vi "BLEGUI.vi"() -> ()   [LabVIEW 2019]
doc: "This example performs writes and reads on a serial port, as directed by the user. You can press the Write and Read buttons, and change the Read Count, while the example is running.\n\nThe parameters set for the serial port must match the parameters of the connected instrument or device. In this example, the Read Count parameter specifies the number of bytes that the serial port reads. If there were more bytes at the port than the specified number, those bytes would not be read. If there were less bytes at the port than the specified number, you would receive a timeout error.\n\nThis example expands upon the flow control options for XON and XOFF, allowing the user to choose those control characters. Also, the user can enable or disable a termination character. Some devices require a termination character in order to identify the end of command strings. Some devices send a termination character to signify the end of data to be read. This example shows how you can end the Read operation once a termination character is detected in the buffer and/or append a termination character at the end of the Write data."
uses:
  Serial - Settings.ctl
  Serial - XON-XOFF Characters.ctl
  Serial - ASCII Characters.ctl
  <vilib>/Instr/_visa.llb/VISA Configure Serial Port (Instr).vi
panel:
  in  "Stop":bool
  in  "Termination Character":u8=10 format="%.0x"
  in  "End Write on Termination Character?":bool=TRUE
  in  "XON/XOFF Characters":T1={"XON"=enum."DC1", "XOFF"=enum."DC3"}
  in  "Serial Settings":T3={"baud rate"=9600, "data bits"=8, "parity"=enum."None", "stop bits"=10, "flow control"=0} {"flow control" items=["None"=0, "XON/XOFF"=1, "RTS/CTS"=2, "DTR/DSR"=4]; "stop bits" items=["1.0"=10, "1.5"=15, "2.0"=20]; "data bits" min=5 max=8 step=1; "baud rate" items=["75"=75, "110"=110, "134"=134, "150"=150, "300"=300, "600"=600, "1200"=1200, "1800"=1800, "2400"=2400, "4800"=4800, "7200"=7200, "9600"=9600, "14400"=14400, "19200"=19200, "28800"=28800, "38400"=38400, "56000"=56000, "57600"=57600, "115200"=115200, "128000"=128000, "230400"=230400]}
  in  "End Read on Termination Character?":bool=TRUE
  in  "VISA resource name":refnum<visa-resource-name>="COM1"
  in  "Read Count":u32=1000
  out "Response":string
  out "Gyro":T4(graph)
  out "Acc":T4(graph)
  out "W4":dbl
  out "W3":dbl
  out "W2":dbl
  out "W1":dbl
  out "GZ":dbl
  out "GY":dbl
  out "GX":dbl
  out "Z":dbl
  out "Y":dbl
  out "X":dbl
  out "Z":dbl(slide) scale=0.0..2.0
  out "Y":dbl(slide) scale=-1.0..1.0
  out "X":dbl(slide) scale=-1.0..1.0
  out "Roll (deg)":dbl(knob) scale=-180.0..180.0
  out "Pitch (deg)":dbl(knob) scale=-90.0..90.0
  in  "Activate Drone Location":bool
  out "Distance 2 (mm)":i32
  out "Ultrasonic 2":dbl(knob) scale=0.0..300.0
  out "Ultrasonic 1":dbl(knob) scale=0.0..300.0
  out "Distance 1 (mm)":i32
  in  "Quick Command":string="*IDN?"
  in  "Command QuadCopter":bool
  in  "Down":bool
  in  "Up":bool
  in  "Left":bool
  in  "Right":bool
  in  "STOP Quadcopter":bool
  # "SERIAL SETTINGS"
  # "0xA is equivalent to a '\\n' character, which is a line feed."
  # "STATUS & CONTINUOUS FEED"
  # "QUADCOPTER & MOTORS"
  # "ON"
  # "OFF"
  # "Speed of Motors (deg s-1)"
  # "Gyro (deg s-1)"
  # "Acc (G)"
  # "MOTION SENSING"
  # "COMMAND QUADCOPTER"
  # "ON"
  # "OFF"
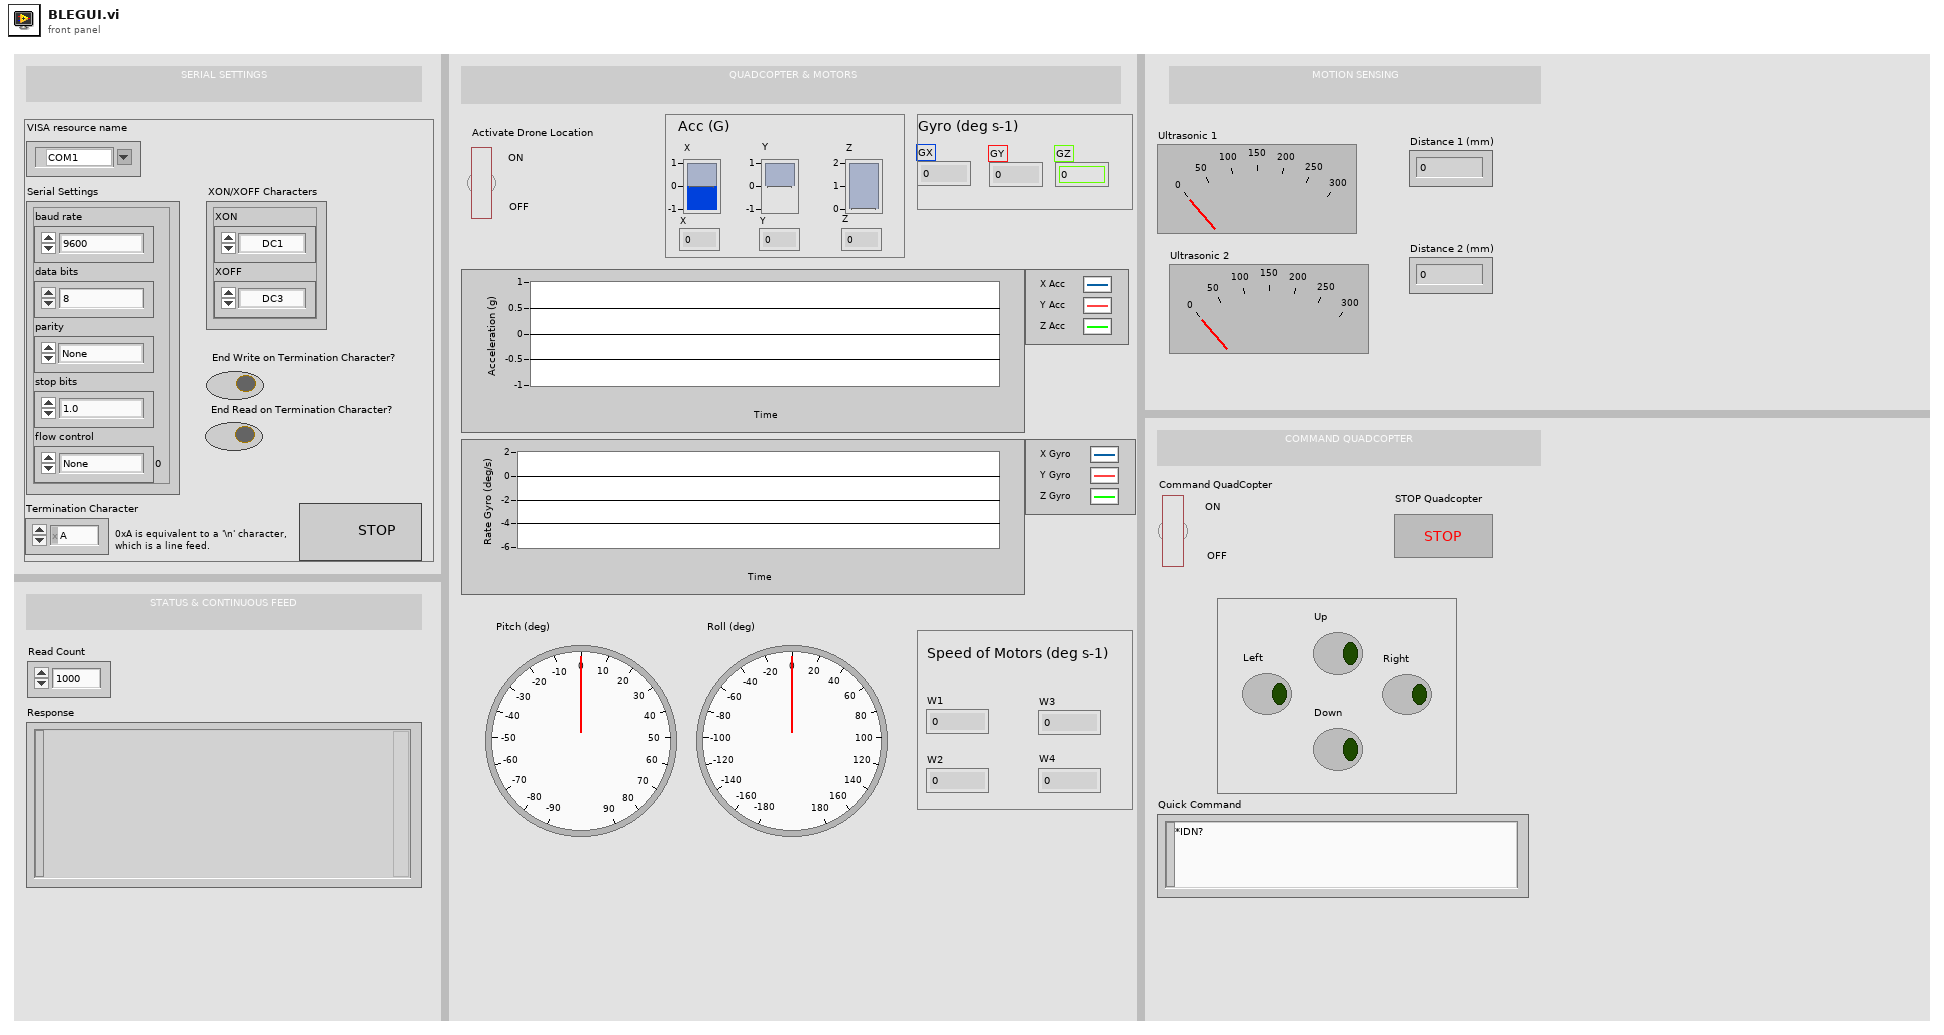
[diagram p1: front panel]
types:
  T1 = typedef "Serial - XON-XOFF Characters.ctl" = cluster{"XON":T2, "XOFF":T2}
  T2 = typedef "Serial - ASCII Characters.ctl" = enum16{"NUL", "SOH", "STX", "ETX", "EOT", "ENQ", "ACK", "BEL", "BS", "HT", "LF", "VT", "FF", "CR", "SO", "SI", "DLE", "DC1", "DC2", "DC3", "DC4", "NAK", "SYN", "ETB", "CAN", "EM", "SUB", "ESC", "FS", "GS", "RS", "US", "SP", "!", "\"", "#", "$", "%", "&", "'", "(", ")", "*", "+", ",", "- (-)", ".", "/", "0", "1", "2", "3", "4", "5", "6", "7", "8", "9", ":", ";", "<", "=", ">", "?", "@", "A", "B", "C", "D", "E", "F", "G", "H", "I", "J", "K", "L", "M", "N", "O", "P", "Q", "R", "S", "T", "U", "V", "W", "X", "Y", "Z", "[", "\\", "]", "^", "_", "`", "a", "b", "c", "d", "e", "f", "g", "h", "i", "j", "k", "l", "m", "n", "o", "p", "q", "r", "s", "t", "u", "v", "w", "x", "y", "z", "{", "|", "}", "~"}
  T3 = typedef "Serial - Settings.ctl" = cluster{"baud rate":u32, "data bits":u16, "parity":enum16{"None", "Odd", "Even", "Mark", "Space"}, "stop bits":u16, "flow control":u16}
  T4 = cluster{"[0]":dbl, "[1]":dbl, "[2]":dbl, "[3]":dbl, "[4]":dbl, "[5]":dbl, "[6]":dbl, "[7]":dbl, "[8]":dbl}
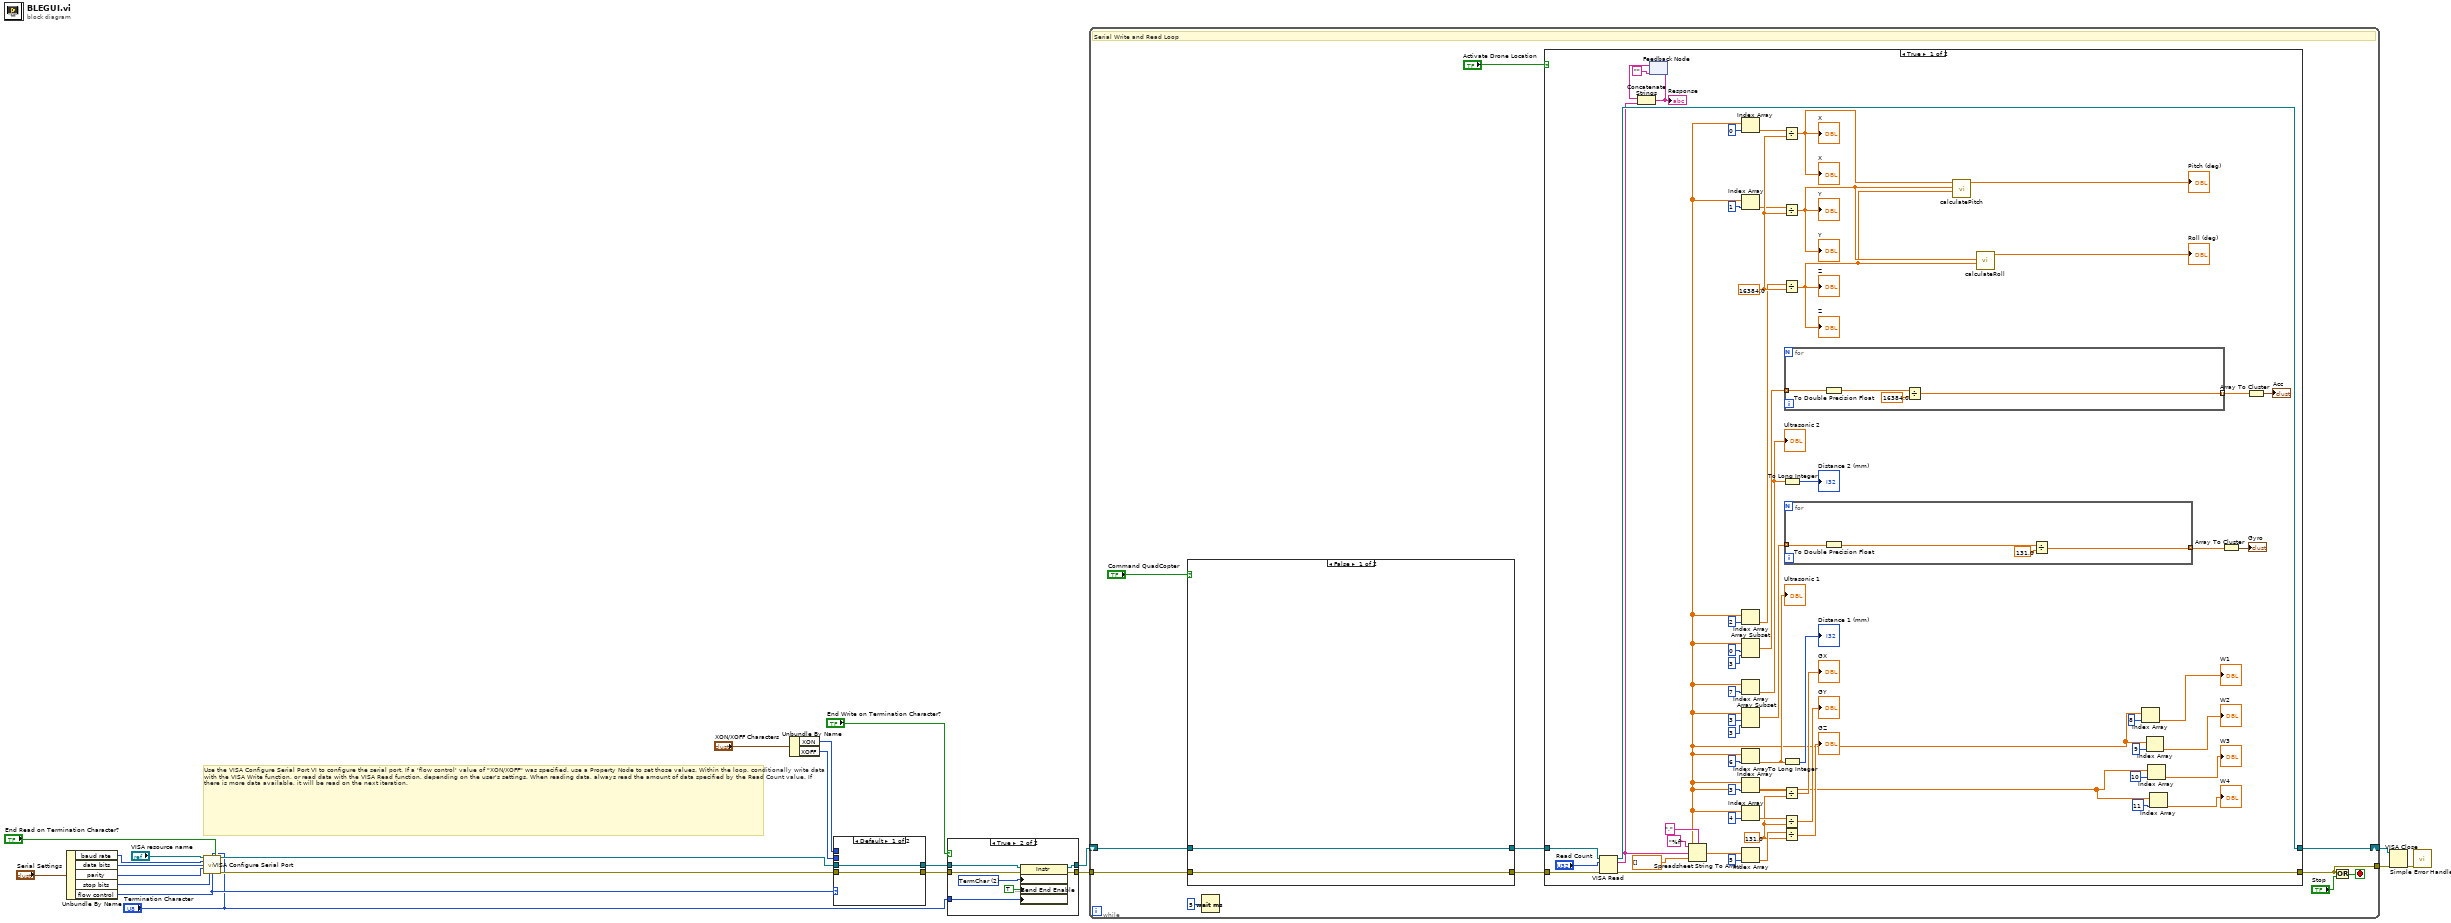
[diagram p0: block diagram]
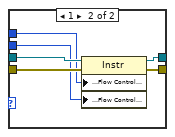
[diagram p3: hidden frame]
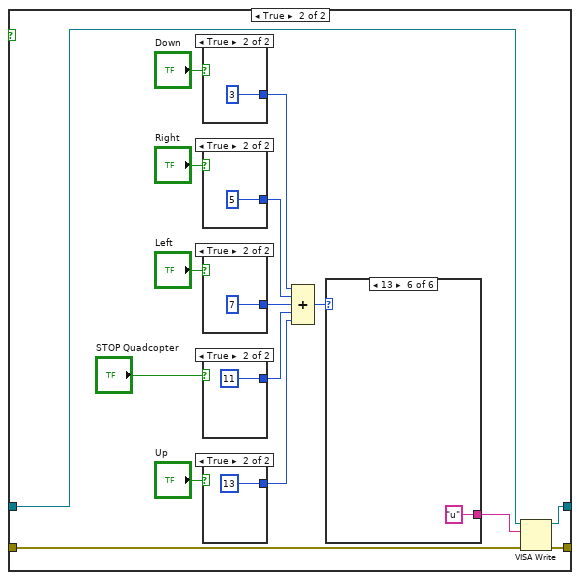
[diagram p4: hidden frame]
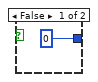
[diagram p5: hidden frame]
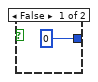
[diagram p6: hidden frame]
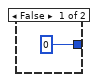
[diagram p7: hidden frame]
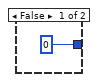
[diagram p8: hidden frame]
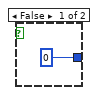
[diagram p9: hidden frame]
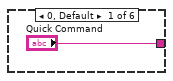
[diagram p10: hidden frame]
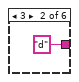
[diagram p11: hidden frame]
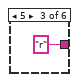
[diagram p12: hidden frame]
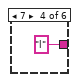
[diagram p13: hidden frame]
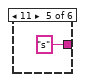
[diagram p14: hidden frame]
diagram:
  # "Use the VISA Configure Serial Port VI to configure the serial port. If a 'flow control' value of \"XON/XOFF\" was specified, use a Property Node to set those values. Within the loop, conditionally write data with the VISA Write function, or read data with the VISA Read function, depending on the user's settings. When reading data, always read the amount of data specified by the Read Count value. If there is more data available, it will be read on the next iteration."
  n1 = Unbundle By Name("Serial Settings") -> ("baud rate"=w15:u32, "data bits"=w16:u16, "parity"=w17:enum16{"None", "Odd", "Even", "Mark", "Space"}, "stop bits"=w18:u16, "flow control"=w9:u16)
  n2 = call-poly "VISA Configure Serial Port"("VISA resource name"="VISA resource name", "termination char\n(0xA = '\\n' = LF)"="Termination Character", "Enable Termination\nChar (T)"="End Read on Termination Character?", "baud rate (9600)"=w15, "data bits (8)"=w16, "parity (0:none)"=w17, "stop bits (10: 1 bit)"=w18, "flow control (0:none)"=w9) -> ("VISA resource name out"=w19:refnum<visa-resource-name>, "error out"=w20:errorcluster)  [unwired: 2 in, 4 out]
  n3 = Unbundle By Name("XON/XOFF Characters") -> ("XON"=w8:T2, "XOFF"=w7:T2)
  n4 = case shown="Default" w9 {
    tunnel: [w23 w30] -> w6
    tunnel: [w24 w29] -> w4
    tunnel: w20 -> [w23 w28]
    tunnel: w19 -> [w24 w27]
    tunnel: w8 -> [_ w26]
    tunnel: w7 -> [_ w25]
    frame Default {
    }
    frame 1 {
      n5 = property class="Instr"(reference=w27, error in=w28, "Serial Settings:Flow Control XON Character"=w26, "Serial Settings:Flow Control XOFF Character"=w25) -> (reference out=w29:refnum<visa-resource-name>, error out=w30:errorcluster)
    }
  }
  n6 = case shown="True" "End Write on Termination Character?" {
    tunnel: w4 -> [w31 w39]
    tunnel: w6 -> [w32 w38]
    tunnel: [w31 w37] -> w3
    tunnel: [w32 w36] -> w5
    tunnel: "Termination Character" -> [_ w34]
    frame False {
    }
    frame True {
      w35 = u16 2 items=["None", "LastBit", "TermChar", "Break"] ("Serial Settings:Serial End Mode for Writes")
      n7 = property class="Instr"(reference=w39, error in=w38, "Serial Settings:End Mode for Writes"=w35, "Message Based Settings:Send End Enable"=TRUE, "Message Based Settings:Termination Character"=w34) -> (reference out=w37:refnum<visa-resource-name>, error out=w36:errorcluster)
    }
  }
  n8 = while {
    shift-right: [w50] -> w10
    shift-left: w3 -> [w49]
    tunnel: w5 -> [w48]
    tunnel: [w42] -> w11
    stop <- w43 stop-if-true
    # "Serial Write and Read Loop"
    n9 = case shown="False" "Command QuadCopter" {
      tunnel: w49 -> [w52 w68]
      tunnel: w48 -> [w51 w67]
      tunnel: [w52 w66] -> w47
      tunnel: [w51 w65] -> w46
      frame False {
      }
      frame True {
        n10 = case shown="True" "Down" {
          tunnel: [0 3] -> w59
          frame False {
          }
          frame True {
          }
        }
        n11 = case shown="True" "Right" {
          tunnel: [0 5] -> w58
          frame False {
          }
          frame True {
          }
        }
        n12 = case shown="True" "Left" {
          tunnel: [0 7] -> w57
          frame False {
          }
          frame True {
          }
        }
        n13 = case shown="True" "STOP Quadcopter" {
          tunnel: [0 11] -> w56
          frame False {
          }
          frame True {
          }
        }
        n14 = case shown="True" "Up" {
          tunnel: [0 13] -> w55
          frame False {
          }
          frame True {
          }
        }
        n15 = Compound Arithmetic op=ADD(w59, w58, w57, w56, w55) -> (w54:i32)
        n16 = case shown="13" w54 {
          tunnel: ["Quick Command" "d" "r" "l" "s" "u"] -> w53
          frame 0, Default {
          }
          frame 3 {
          }
          frame 5 {
          }
          frame 7 {
          }
          frame 11 {
          }
          frame 13 {
          }
        }
        n17 = VISA Write(VISA resource name=w68, write buffer=w53, error in (no error)=w67) -> (VISA resource name out=w66:refnum<visa-resource-name>, error out=w65:errorcluster)  [unwired: 1 out]
      }
    }
    n18 = Wait (ms)(milliseconds to wait=u32 5) -> ()  [unwired: 1 out]
    n19 = case shown="True" "Activate Drone Location" {
      tunnel: [w141 w153] -> w50
      tunnel: w47 -> [w143 w153]
      tunnel: [w139 w152] -> w42
      tunnel: w46 -> [w142 w152]
      frame True {
        w119 = 131.0 ("y")
        w128 = 16384.0 ("y")
        n20 = VISA Read(VISA resource name=w143, byte count="Read Count", error in (no error)=w142) -> (VISA resource name out=w141:refnum<visa-resource-name>, read buffer=w118:string, error out=w139:errorcluster)  [unwired: 1 out]
        n21 = feedback #1("") -> (w138:string)
        n22 = Concatenate Strings(w138, w118) -> (w136:string)
        "Response" <- w136
        n23 = feedback-in #1(w136) -> ()
        n24 = Spreadsheet String To Array(delimiter (Tab)=",", format string="%f", spreadsheet string=w118, array type (2D Dbl)=dbl[] []) -> (array=w85:dbl[])
        n25 = Index Array(array=w85, index=0) -> (element=w129:dbl)
        n26 = Index Array(array=w85, index=1) -> (element=w126:dbl)
        n27 = Index Array(array=w85, index=2) -> (element=w127:dbl)
        n28 = Array Subset(array=w85, index=0, length=3) -> (w101:dbl[])
        n29 = Index Array(array=w85, index=7) -> (element=w110:dbl)
        "Ultrasonic 2" <- w110
        n30 = Array Subset(array=w85, index=3, length=3) -> (w98:dbl[])
        n31 = Index Array(array=w85, index=6) -> (element=w113:dbl)
        "Ultrasonic 1" <- w113
        n32 = Index Array(array=w85, index=3) -> (element=w122:dbl)
        n33 = Index Array(array=w85, index=4) -> (element=w121:dbl)
        n34 = Index Array(array=w85, index=5) -> (element=w120:dbl)
        n35 = Divide(x=w129, y=w128) -> (x/y=w106:dbl)
        "X" <- w106
        "X" <- w106
        n36 = Divide(x=w126, y=w128) -> (x/y=w105:dbl)
        "Y" <- w105
        "Y" <- w105
        n37 = Divide(x=w127, y=w128) -> (x/y=w104:dbl)
        "Z" <- w104
        "Z" <- w104
        n38 = To Long Integer(number=w110) -> (32bit integer=→"Distance 2 (mm)":i32)
        n39 = To Long Integer(number=w113) -> (32bit integer=→"Distance 1 (mm)":i32)
        n40 = Divide(x=w122, y=w119) -> (x/y=→"GX":dbl)
        n41 = Divide(x=w121, y=w119) -> (x/y=→"GY":dbl)
        n42 = Divide(x=w120, y=w119) -> (x/y=→"GZ":dbl)
        n43 = for {
          tunnel: w101 -> [w151] mode=indexing
          tunnel: [w148] -> w100 mode=indexing
          n44 = To Double Precision Float(number=w151) -> (double precision float=w150:dbl)
          n45 = Divide(x=w150, y=16384.0) -> (x/y=w148:dbl)
        }
        n46 = for {
          tunnel: w98 -> [w147] mode=indexing
          tunnel: [w144] -> w99 mode=indexing
          n47 = To Double Precision Float(number=w147) -> (double precision float=w146:dbl)
          n48 = Divide(x=w146, y=131.0) -> (x/y=w144:dbl)
        }
        n49 = call "calculatePitch.vi"("az"=w104, "ay"=w105, "ax"=w106) -> ("pitch"=→"Pitch (deg)":dbl)  [unwired: 8 in]
        n50 = call "calculateRoll.vi"("az"=w104, "ay"=w105) -> ("roll"=→"Roll (deg)":dbl)  [unwired: 9 in]
        n51 = Index Array(array=w85, index=8) -> (element=→"W1":dbl)
        n52 = Index Array(array=w85, index=9) -> (element=→"W2":dbl)
        n53 = Index Array(array=w85, index=10) -> (element=→"W3":dbl)
        n54 = Index Array(array=w85, index=11) -> (element=→"W4":dbl)
        n55 = Array To Cluster(array=w99) -> (cluster=→"Gyro":T4)
        n56 = Array To Cluster(array=w100) -> (cluster=→"Acc":T4)
      }
      frame False {
      }
    }
    n57 = Or(x=w42, y="Stop") -> (x .or. y?=w43:bool)
  }
  n58 = VISA Close(VISA resource name=w10, error in (no error)=w11) -> (error out=w12:errorcluster)
  n59 = call <vilib>:"Simple Error Handler.vi"("error in (no error)"=w12) -> ()  [unwired: 1 in, 8 out]
